vi "VarB.vi"(2 "RCW (X2)":dbl(slide) scale=-1.0..1.0, 3 "STR (X)":dbl(slide) scale=-1.0..1.0, 4 "R":dbl, 5 "L":dbl) -> (0 "B = 0?":bool, 1 "B":dbl)   [LabVIEW 2012]
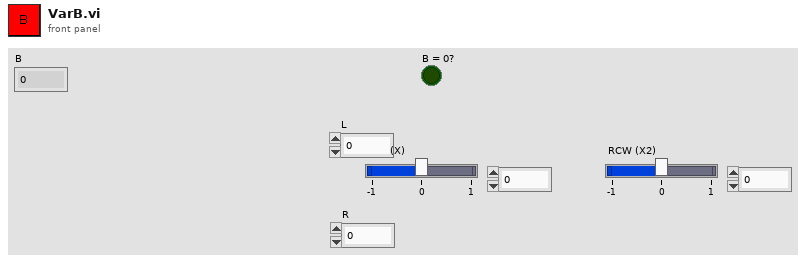
[diagram p1: front panel]
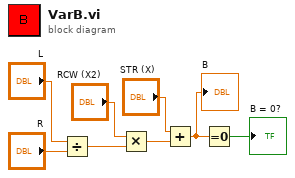
[diagram p0: block diagram]
diagram:
  n1 = Divide(x="L", y="R") -> (x/y=w5:dbl)
  n2 = Multiply(x="RCW (X2)", y=w5) -> (x*y=w3:dbl)
  n3 = Add(x="STR (X)", y=w3) -> (x+y=w2:dbl)
  "B" <- w2
  n4 = Equal To 0?(x=w2) -> (x = 0?=→"B = 0?":bool)
